vi "HXG2_SelectDataToPlot.vi"(7 "Plot Selection":u16[](array[ring]), 8 "error IO":errorcluster, 11 "Numeric Array In":dbl[](array[numeric])) -> (0 "error Out":errorcluster, 3 "Array of Waveform Out":waveform(dbl)[](array[waveform]))   [LabVIEW 2012]
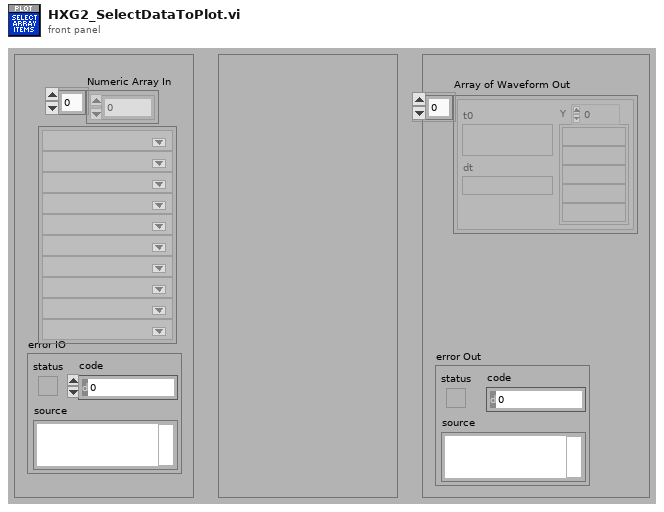
[diagram p1: front panel]
types:
  T1 = cluster{"[0]":dbl, "[1]":dbl, "[2]":dbl, "[3]":dbl, "[4]":dbl, "[5]":dbl, "[6]":dbl, "[7]":dbl, "[8]":dbl, "[9]":dbl}
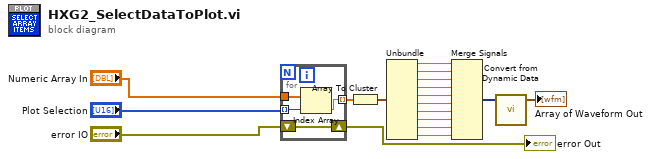
[diagram p0: block diagram]
diagram:
  n1 = for {
    tunnel: [w22] -> w18 mode=indexing
    shift-right: [w21] -> w7
    shift-left: "error IO" -> [w21]
    tunnel: "Numeric Array In" -> [w20]
    tunnel: "Plot Selection" -> [w19] mode=indexing
    n2 = Index Array(array=w20, index=w19) -> (element=w22:dbl)
  }
  "error Out" <- w7
  n3 = Array To Cluster(array=w18) -> (cluster=w6:T1)
  n4 = Unbundle(w6) -> ("[0]"=w8:dbl, "[1]"=w9:dbl, "[2]"=w10:dbl, "[3]"=w11:dbl, "[4]"=w12:dbl, "[5]"=w13:dbl, "[6]"=w14:dbl, "[7]"=w15:dbl, "[8]"=w16:dbl, "[9]"=w17:dbl)
  n5 = Merge Signals(w8, w9, w10, w11, w12, w13, w14, w15, w16, w17) -> (w3:dynamicdata)
  n6 = call "Convert from Dynamic Data"("Dynamic Data Type"=w3) -> ("Array of Waveform"=→"Array of Waveform Out":waveform(dbl)[])  [unwired: 3 in]
